vi "create lines.vi"(0 "HarpDataFrame":T3, 2 "use system decimal point (T)":bool, 7 "EnableList":T2={"Cmd"=FALSE, "RegAdd"=FALSE, "Port"=FALSE, "Rsvd"=FALSE, "UTC"=FALSE, "Error"=FALSE, "Type"=FALSE, "NElements"=FALSE, "BitElementsColumn"=FALSE, "BitElementsAtTheEnd"=FALSE, "Read"=TRUE, "Write"=TRUE, "Event"=TRUE, "No Errors"=FALSE}, 12 "Filter:":T1(ring), 13 "List:":string) -> (8 "Line":string)   [LabVIEW 2010]
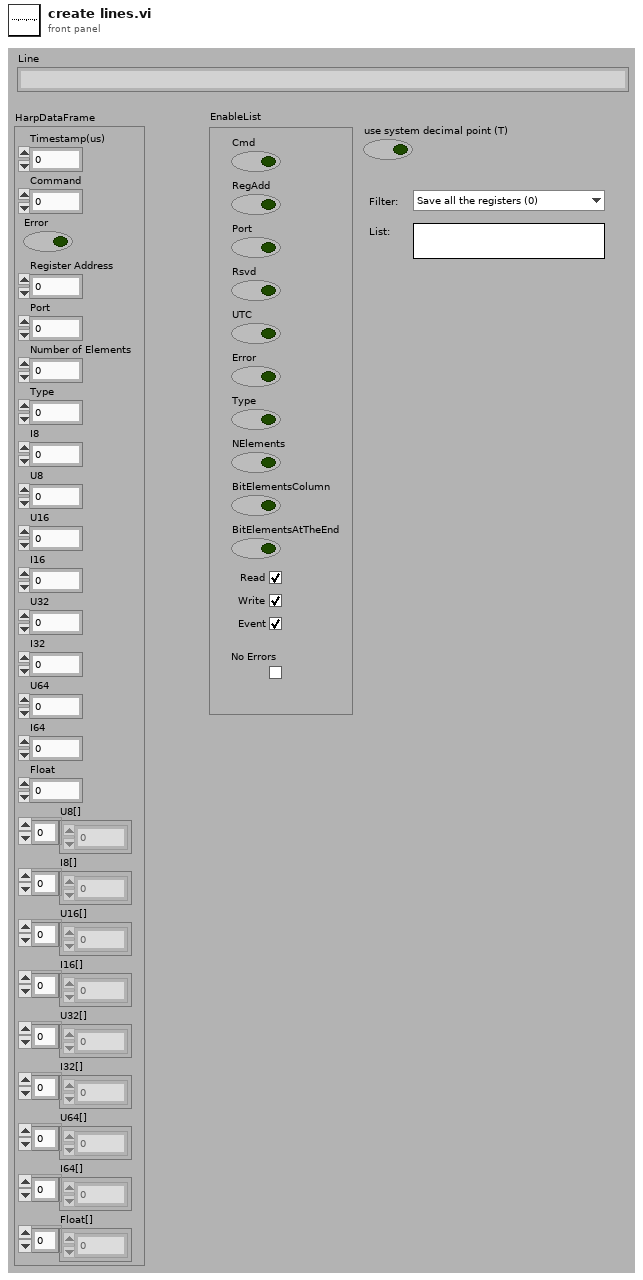
[diagram p1: front panel]
types:
  T1 = enum16{"Save all the registers (0)", "Save only specific registers (1)"}
  T2 = cluster{"Cmd":bool, "RegAdd":bool, "Port":bool, "Rsvd":bool, "UTC":bool, "Error":bool, "Type":bool, "NElements":bool, "BitElementsColumn":bool, "BitElementsAtTheEnd":bool, "Read":bool, "Write":bool, "Event":bool, "No Errors":bool}
  T3 = cluster{"Timestamp(us)":dbl, "Command":u8, "Error":bool, "Register Address":u8, "Port":u8, "Number of Elements":u8, "Type":u8, "I8":i8, "U8":u8, "U16":u16, "I16":i16, "U32":u32, "I32":i32, "U64":u64, "I64":i64, "Float":sgl, "U8[]":u8[], "I8[]":i8[], "U16[]":u16[], "I16[]":i16[], "U32[]":u32[], "I32[]":i32[], "U64[]":u64[], "I64[]":i64[], "Float[]":sgl[]}
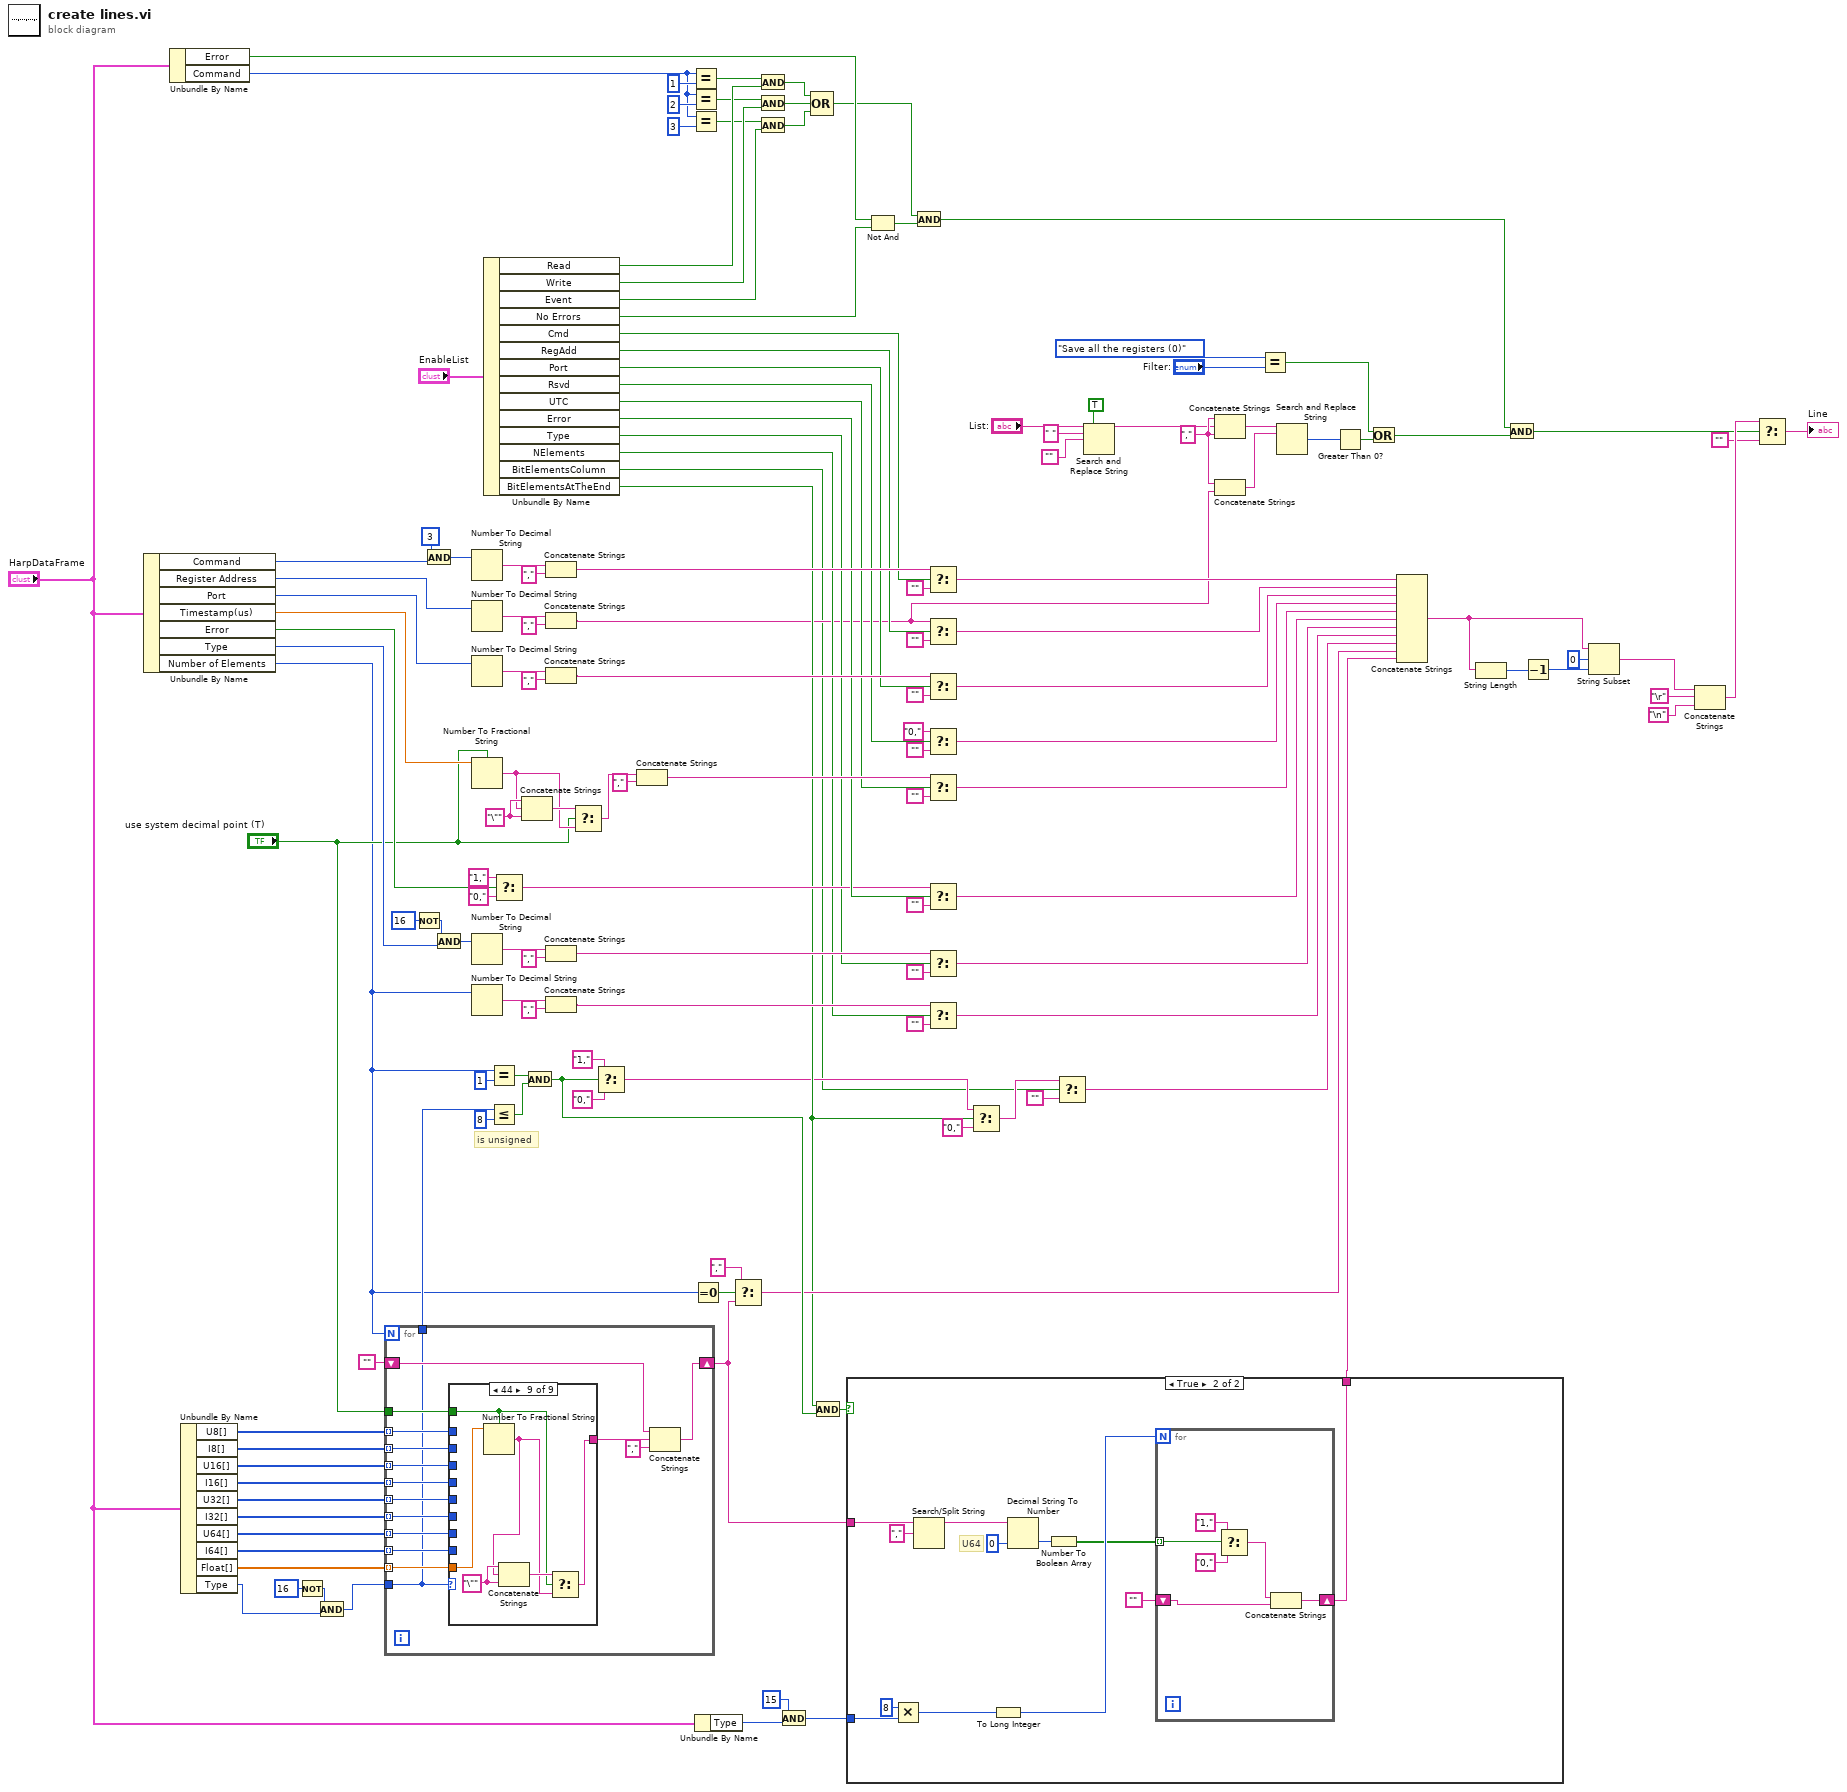
[diagram p0: block diagram]
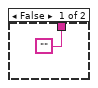
[diagram p2: hidden frame]
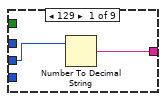
[diagram p3: hidden frame]
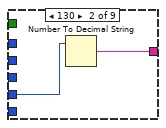
[diagram p4: hidden frame]
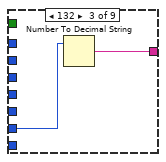
[diagram p5: hidden frame]
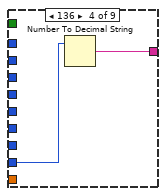
[diagram p6: hidden frame]
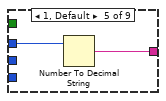
[diagram p7: hidden frame]
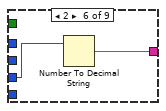
[diagram p8: hidden frame]
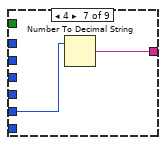
[diagram p9: hidden frame]
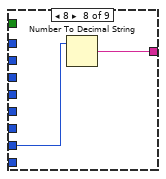
[diagram p10: hidden frame]
diagram:
  w13 = "," ("string")
  w69 = "\"" ("string")
  # "is unsigned"
  n1 = Unbundle By Name("HarpDataFrame") -> ("Command"=w145:u8, "Register Address"=w138:u8, "Port"=w137:u8, "Timestamp(us)"=w119:dbl, "Error"=w113:bool, "Type"=w104:u8, "Number of Elements"=w25:u8)
  n2 = Unbundle By Name("HarpDataFrame") -> ("Error"=w44:bool, "Command"=w34:u8)
  n3 = Unbundle By Name("HarpDataFrame") -> ("U8[]"=w97:u8[], "I8[]"=w96:i8[], "U16[]"=w95:u16[], "I16[]"=w94:i16[], "U32[]"=w93:u32[], "I32[]"=w92:i32[], "U64[]"=w91:u64[], "I64[]"=w90:i64[], "Float[]"=w89:sgl[], "Type"=w77:u8)
  n4 = Not(x=u8 16) -> (.not. x?=w80:u8)
  n5 = And(x=w80, y=w77) -> (x .and. y?=w78:u8)
  n6 = for {
    N: w25 -> [_]
    tunnel: w97 -> [w160] mode=indexing
    tunnel: w96 -> [w151] mode=indexing
    tunnel: w95 -> [w155] mode=indexing
    tunnel: w94 -> [w150] mode=indexing
    tunnel: w93 -> [w154] mode=indexing
    tunnel: w92 -> [w149] mode=indexing
    tunnel: w91 -> [w153] mode=indexing
    tunnel: w90 -> [w148] mode=indexing
    tunnel: w89 -> [w152] mode=indexing
    tunnel: w78 -> [w146]
    shift-right: [w156] -> w21
    shift-left: "" -> [w157]
    tunnel: "use system decimal point (T)" -> [w147]
    tunnel: [w146] -> w50
    n7 = case shown="44" w146 {
      tunnel: w160 -> [_ _ _ _ w170 _ _ _ _]
      tunnel: [w162 w164 w166 w168 w169 w172 w174 w176 w178] -> w158
      tunnel: w155 -> [_ _ _ _ _ w171 _ _ _]
      tunnel: w154 -> [_ _ _ _ _ _ w173 _ _]
      tunnel: w153 -> [_ _ _ _ _ _ _ w175 _]
      tunnel: w152 -> [_ _ _ _ _ _ _ _ w182]
      tunnel: w151 -> [w161 _ _ _ _ _ _ _ _]
      tunnel: w150 -> [_ w163 _ _ _ _ _ _ _]
      tunnel: w149 -> [_ _ w165 _ _ _ _ _ _]
      tunnel: w148 -> [_ _ _ w167 _ _ _ _ _]
      tunnel: w147 -> [_ _ _ _ _ _ _ _ w177]
      frame 129 {
        n8 = Number To Decimal String(number=w161) -> (decimal integer string=w162:string)  [unwired: 1 in]
      }
      frame 130 {
        n9 = Number To Decimal String(number=w163) -> (decimal integer string=w164:string)  [unwired: 1 in]
      }
      frame 132 {
        n10 = Number To Decimal String(number=w165) -> (decimal integer string=w166:string)  [unwired: 1 in]
      }
      frame 136 {
        n11 = Number To Decimal String(number=w167) -> (decimal integer string=w168:string)  [unwired: 1 in]
      }
      frame 1, Default {
        n12 = Number To Decimal String(number=w170) -> (decimal integer string=w169:string)  [unwired: 1 in]
      }
      frame 2 {
        n13 = Number To Decimal String(number=w171) -> (decimal integer string=w172:string)  [unwired: 1 in]
      }
      frame 4 {
        n14 = Number To Decimal String(number=w173) -> (decimal integer string=w174:string)  [unwired: 1 in]
      }
      frame 8 {
        n15 = Number To Decimal String(number=w175) -> (decimal integer string=w176:string)  [unwired: 1 in]
      }
      frame 68 {
        w180 = "\"" ("string")
        n16 = Number To Fractional String(use system decimal point (T)=w177, number=w182) -> (F-format string=w179:string)  [unwired: 2 in]
        n17 = Concatenate Strings(w180, w179, w180) -> (w181:string)
        n18 = Select(t=w181, s=w177, f=w179) -> (s? t:f=w178:string)
      }
    }
    n19 = Concatenate Strings(w157, w158, "," ("string")) -> (w156:string)
  }
  n20 = Not(x=u8 16) -> (.not. x?=w105:u8)
  n21 = And(x=u8 3, y=w145) -> (x .and. y?=w143:u8)
  n22 = And(x=w105, y=w104) -> (x .and. y?=w107:u8)
  n23 = Number To Decimal String(number=w143) -> (decimal integer string=w142:string)  [unwired: 1 in]
  n24 = Number To Decimal String(number=w138) -> (decimal integer string=w131:string)  [unwired: 1 in]
  n25 = Number To Decimal String(number=w137) -> (decimal integer string=w130:string)  [unwired: 1 in]
  n26 = Number To Fractional String(use system decimal point (T)="use system decimal point (T)", number=w119) -> (F-format string=w67:string)  [unwired: 2 in]
  n27 = Number To Decimal String(number=w107) -> (decimal integer string=w108:string)  [unwired: 1 in]
  n28 = Number To Decimal String(number=w25) -> (decimal integer string=w102:string)  [unwired: 1 in]
  n29 = Unbundle By Name("EnableList") -> ("Read"=w41:bool, "Write"=w38:bool, "Event"=w37:bool, "No Errors"=w45:bool, "Cmd"=w128:bool, "RegAdd"=w127:bool, "Port"=w126:bool, "Rsvd"=w124:bool, "UTC"=w118:bool, "Error"=w116:bool, "Type"=w103:bool, "NElements"=w98:bool, "BitElementsColumn"=w7:bool, "BitElementsAtTheEnd"=w16:bool)
  n30 = Equal?(x=w25, y=u8 1) -> (x = y?=w55:bool)
  n31 = Less Or Equal?(x=w50, y=u8 8) -> (x <= y?=w49:bool)
  n32 = Select(t="1," ("string"), s=w113, f="0,") -> (s? t:f=w112:string)
  n33 = Concatenate Strings(w69, w67, w69) -> (w68:string)
  n34 = And(x=w55, y=w49) -> (x .and. y?=w47:bool)
  n35 = Concatenate Strings(w142, "," ("string")) -> (w136:string)
  n36 = Concatenate Strings(w131, "," ("string")) -> (w14:string)
  n37 = Concatenate Strings(w130, "," ("string")) -> (w132:string)
  n38 = Concatenate Strings(w108, "," ("string")) -> (w110:string)
  n39 = Concatenate Strings(w102, "," ("string")) -> (w101:string)
  n40 = Select(t=w68, s="use system decimal point (T)", f=w67) -> (s? t:f=w66:string)
  n41 = Select(t="1," ("string"), s=w47, f="0," ("string")) -> (s? t:f=w8:string)
  n42 = Concatenate Strings(w66, "," ("string")) -> (w122:string)
  n43 = Equal?(x=w34, y=u8 1) -> (x = y?=w42:bool)
  n44 = Equal?(x=w34, y=u8 2) -> (x = y?=w40:bool)
  n45 = Equal?(x=w34, y=u8 3) -> (x = y?=w35:bool)
  n46 = Equal To 0?(x=w25) -> (x = 0?=w24:bool)
  n47 = Unbundle By Name("HarpDataFrame") -> ("Type"=w20:u8)
  n48 = Select(t="," ("string"), s=w24, f=w21) -> (s? t:f=w22:string)
  n49 = And(x=w42, y=w41) -> (x .and. y?=w33:bool)
  n50 = And(x=w40, y=w38) -> (x .and. y?=w32:bool)
  n51 = And(x=w35, y=w37) -> (x .and. y?=w31:bool)
  n52 = And(x=u8 15, y=w20) -> (x .and. y?=w17:u8)
  n53 = Compound Arithmetic op=OR(w33, w32, w31) -> (w29:bool)
  n54 = And(x=w16, y=w47) -> (x .and. y?=w48:bool)
  n55 = case shown="True" w48 {
    tunnel: ["" w184] -> w46
    tunnel: w21 -> [_ w195]
    tunnel: w17 -> [_ w191]
    frame False {
    }
    frame True {
      # "U64"
      n56 = Multiply(x=u8 8, y=w191) -> (x*y=w188:u8)
      n57 = Search/Split String(string=w195, search string/char (-)="," ("search string")) -> (substring before match=w193:string)  [unwired: 1 in, 2 out]
      n58 = To Long Integer(number=w188) -> (32bit integer=w187:i32)
      n59 = Decimal String To Number(string=w193, default (0L)=u64 0 ("default (0 I32)")) -> (number=w189:u64)  [unwired: 1 in, 1 out]
      n60 = Number To Boolean Array(number=w189) -> (Boolean array=w186:bool[])
      n61 = for {
        N: w187 -> [_]
        tunnel: w186 -> [w199] mode=indexing
        shift-right: [w197] -> w184
        shift-left: "" -> [w196]
        n62 = Select(t="1," ("string"), s=w199, f="0," ("string")) -> (s? t:f=w198:string)
        n63 = Concatenate Strings(w198, w196) -> (w197:string)
      }
    }
  }
  n64 = Not And(1:w45, 2:w44) -> (0:w30:bool)
  n65 = And(x=w29, y=w30) -> (x .and. y?=w27:bool)
  n66 = Select(t=w136, s=w128, f="") -> (s? t:f=w87:string)
  n67 = Select(t=w14, s=w127, f="") -> (s? t:f=w64:string)
  n68 = Select(t=w132, s=w126, f="") -> (s? t:f=w86:string)
  n69 = Select(t="0," ("string"), s=w124, f="") -> (s? t:f=w85:string)
  n70 = Select(t=w122, s=w118, f="") -> (s? t:f=w84:string)
  n71 = Select(t=w112, s=w116, f="") -> (s? t:f=w83:string)
  n72 = Select(t=w110, s=w103, f="") -> (s? t:f=w82:string)
  n73 = Select(t=w101, s=w98, f="") -> (s? t:f=w81:string)
  n74 = Select(t=w8, s=w16, f="0," ("string")) -> (s? t:f=w11:string)
  n75 = Select(t=w11, s=w7, f="") -> (s? t:f=w10:string)
  n76 = Search and Replace String(replace all?=TRUE ("replace all? (F)"), input string="List:", search string=" ", replace string="") -> (result string=w2:string)  [unwired: 4 in, 3 out]
  n77 = Concatenate Strings(w13, w2, w13) -> (w56:string)
  n78 = Concatenate Strings(w13, w14) -> (w12:string)
  n79 = Equal?(x=T1."Save all the registers (0)", y="Filter:") -> (x = y?=w59:bool)
  n80 = Search and Replace String(input string=w56, search string=w12) -> (number of replacements=w63:i32)  [unwired: 6 in, 3 out]
  n81 = Greater Than 0?(x=w63) -> (x > 0?=w60:bool)
  n82 = Or(x=w59, y=w60) -> (x .or. y?=w28:bool)
  n83 = Concatenate Strings(w87, w64, w86, w85, w84, w83, w82, w81, w10, w22, w46) -> (w73:string)
  n84 = String Length(string=w73) -> (length=w76:i32)
  n85 = And(x=w27, y=w28) -> (x .and. y?=w26:bool)
  n86 = Decrement(x=w76) -> (x-1=w74:i32)
  n87 = String Subset(string=w73, offset (0)=0, length (rest)=w74) -> (substring=w70:string)
  n88 = Concatenate Strings(w70, "\r", "\n") -> (w58:string)
  n89 = Select(t=w58, s=w26, f="") -> (s? t:f=→"Line":string)
